vi "FpgaLink_Scan_Chain.vi"(6 "# of Devices to Return (8)":u32=8, 8 "error in (no error)":errorcluster, 11 "handle":i64) -> (0 "error out":errorcluster, 1 "Number of Devices":u32, 2 "Devices":u32[](array[numeric]), 3 "handle out":i64)   [LabVIEW 2011]
doc: "Scan the JTAG chain and return an array of IDCODEs.\n\nCount the number of devices on the JTAG chain, and set *numDevices accordingly. Then, if deviceArray is not NULL, populate it with at most arraySize IDCODEs, in chain order."
uses:
  <vilib>/Utility/importsl/GetValueByPointer/datatype.ctl
  <vilib>/Utility/importsl/GetValueByPointer/GetValueByPointer.xnode
  resource/lvimptsl.dll
  libfpgalink.dll
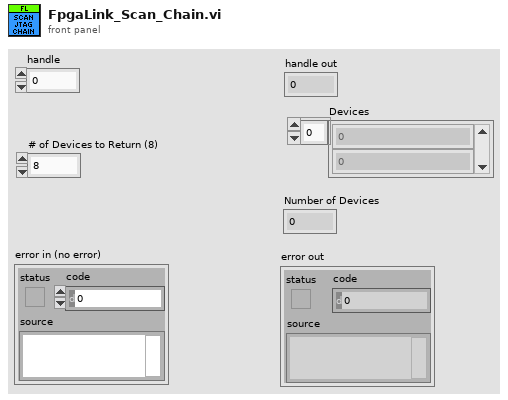
[diagram p1: front panel]
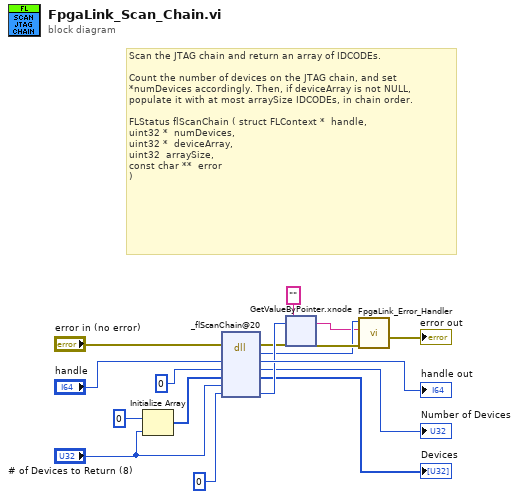
[diagram p0: block diagram]
diagram:
  # "Scan the JTAG chain and return an array of IDCODEs.\n\nCount the number of devices on the JTAG chain, and set *numDevices accordingly. Then, if deviceArray is not NULL, populate it with at most arraySize IDCODEs, in chain order.\n\nFLStatus flScanChain\t(\tstruct FLContext * \thandle,\nuint32 * \tnumDevices,\nuint32 * \tdeviceArray,\nuint32 \tarraySize,\nconst char ** \terror \n)"
  n1 = Initialize Array(u32 0 ("numDevices"), "# of Devices to Return (8)") -> (w4:u32[])
  n2 = dll-call lib="libfpgalink.*" fn="_flScanChain@20"(error in="error in (no error)", "handle"="handle", "numDevices"=u32 0, "deviceArray"=w4, "arraySize"="# of Devices to Return (8)", "error"=i64 0) -> (error out=w12:errorcluster, "FLStatus"=w9:u32, "handle"=→"handle out":i64, "numDevices"=→"Number of Devices":u32, "deviceArray"=→"Devices":u32[], "error"=w13:i64)  [unwired: 3 in, 1 out]
  n3 = xnode "GetValueByPointer.xnode"("Pointer"=w13, "InputType"="", "ErrorIn"=w12) -> ("Output"=w1:string, "ErrorOut"=w10:errorcluster)  [unwired: 1 in]
  n4 = call <vilib>:"FpgaLink_Error_Handler.vi"("error in (no error)"=w10, "error string"=w1, "error code"=w9) -> ("error out"=→"error out":errorcluster)  [unwired: 8 in]
